vi "ClimberDeploy.vi"(8 "error in (no error)":errorcluster, 9 "Deploy/Retract":bool, 10 "Screw":dbl, 11 "ScissorClimber in":refnum<class "ScissorClimber.lvclass">) -> (0 "error out":errorcluster, 3 "ScissorClimber out":refnum<class "ScissorClimber.lvclass">)   [LabVIEW 2019, in "Climber.lvlib" / "ScissorClimber.lvclass"]
uses:
  ScissorClimber.lvclass
  Controls/DeployingStates.ctl
  <vilib>/Rock Robotics/WPI/ThirdParty/Phoenix-LabVIEW/Motor Controller/Controls/CTRE_Phoenix_MotorControl_ControlMode.ctl
  <vilib>/Rock Robotics/WPI/ThirdParty/Phoenix-LabVIEW/Motor Controller/Get/CTRE_Phoenix_MotorController_GetSelectedSensorData.vi
  Climber.lvclass
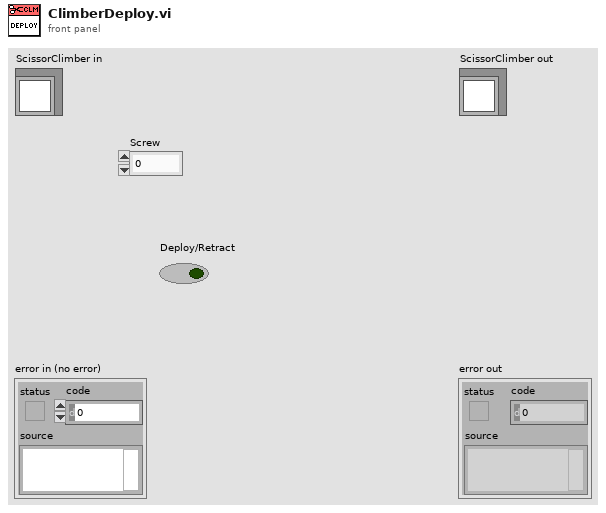
[diagram p1: front panel]
types:
  T1 = typedef "Climber.lvlib/Climber.lvclass/DeployingStates.ctl" = enum16{"Retract", "Manual Control", "Deploying", "Idle"}
  T2 = typedef "Climber.lvlib/Climber.lvclass/Screw Motor.ctl" = cluster{"Refnum Name":string, "CAN ID":u32, "I":dbl, "D":dbl, "P":dbl, "F":dbl, "Velocity":dbl, "Acceleration":dbl}
  T3 = typedef "CTRE_Phoenix_MotorControl_ControlMode.ctl" = u16
  T4 = typedef "WPI_MotorControlDeviceRef.ctl" = cluster{"DeviceStatus":errorcluster, "Type":T5, "PWM":cluster{"PWM Channel":T6, "DeadBand":T7}, "CAN":cluster{"Device Number":u8, "SetOutput VI Ref":variant, "GetOutput VI Ref":variant, "Enable VI Ref":variant, "Disable VI Ref":variant, "Data":variant}, "Invert":bool, "DIO PWM":cluster{"PWM \"Enable\" Channel":T6, "DIOChannel":T8, "PWM Rate":dbl}}
  T5 = typedef "WPI_MotorControlType.ctl" = enum16{"PWM", "CAN", "DIO PWM"}
  T6 = typedef "FPGA_DIOPWMChannel.ctl" = enum8{"PWM 0", "PWM 1", "PWM 2", "PWM 3", "PWM 4", "PWM 5", "PWM 6", "PWM 7", "PWM 8", "PWM 9", "PWM MXP 0", "PWM MXP 1", "PWM MXP 2", "PWM MXP 3", "PWM MXP 4", "PWM MXP 5", "PWM MXP 6", "PWM MXP 7", "PWM MXP 8", "PWM MXP 9", "Invalid"}
  T7 = typedef "WPI_PWMDeadband.ctl" = cluster{"Name":string, "maxPositivePwm":i32, "minPositivePwm":i32, "centerPwm":i32, "maxNegativePwm":i32, "minNegativePwm":i32, "angularRange":u16}
  T8 = typedef "FPGA_DIOChannel.ctl" = enum8{"DIO 0", "DIO 1", "DIO 2", "DIO 3", "DIO 4", "DIO 5", "DIO 6", "DIO 7", "DIO 8", "DIO 9", "DIO MXP 0", "DIO MXP 1", "DIO MXP 2", "DIO MXP 3", "DIO MXP 4", "DIO MXP 5", "DIO MXP 6", "DIO MXP 7", "DIO MXP 8", "DIO MXP 9", "DIO MXP 10", "DIO MXP 11", "DIO MXP 12", "DIO MXP 13", "DIO MXP 14", "DIO MXP 15", "SPI Port CS1", "SPI Port CS2", "SPI Port CS3", "SPI Port MISO", "SPI Port MOSI", "Invalid"}
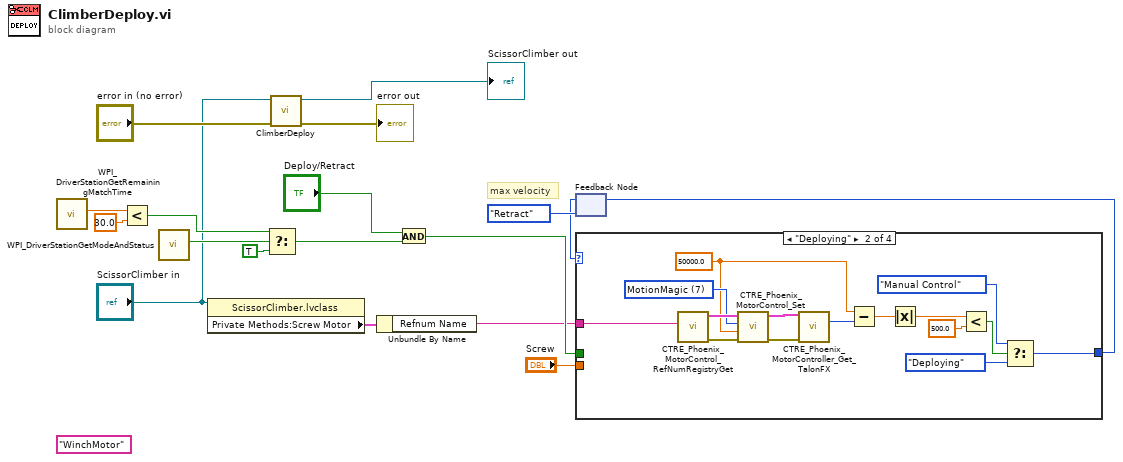
[diagram p0: block diagram]
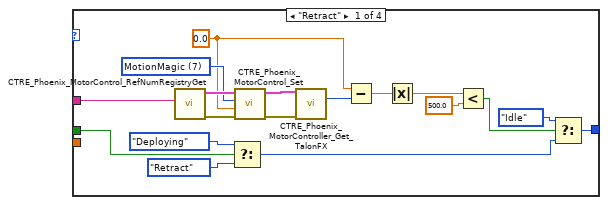
[diagram p2: hidden frame]
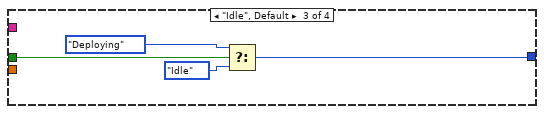
[diagram p3: hidden frame]
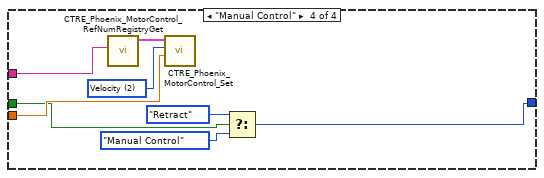
[diagram p4: hidden frame]
diagram:
  (unwired) "WinchMotor"
  # "max velocity"
  n1 = call <vilib>:"WPI_DriverStationGetRemainingMatchTime.vi"() -> ("Match Time(s)"=w15:sgl)  [unwired: 10 in, 1 out]
  n2 = Less?(x=w15, y=30.0) -> (x < y?=w11:bool)
  n3 = call <vilib>:"WPI_DriverStationGetModeAndStatus.vi"() -> ("FMS Attached"=w13:bool)  [unwired: 10 in, 1 out]
  n4 = property class="ScissorClimber.lvclass"(reference="ScissorClimber in") -> ("Private Methods:Screw Motor"=w2:T2)  [unwired: 1 in, 2 out]
  n5 = Select(t=w11, s=w13, f=TRUE) -> (s? t:f=w10:bool)
  n6 = call-parent "ClimberDeploy.vi"("error in (no error)"="error in (no error)", "Climber in"="ScissorClimber in") -> ("error out"=→"error out":errorcluster, "Climber out"=→"ScissorClimber out":refnum<class "ScissorClimber.lvclass">)  [unwired: 8 in]
  n7 = Unbundle By Name(w2) -> ("Refnum Name"=w1:string)
  n8 = And(x="Deploy/Retract", y=w10) -> (x .and. y?=w5:bool)
  n9 = feedback #1(DeployingStates."Retract") -> (w7:T1)
  n10 = case shown="\"Deploying\"" w7 {
    tunnel: [w23 w39 w53 w60] -> w6
    tunnel: w5 -> [w20 _ w52 w59]
    tunnel: "Screw" -> [_ _ _ w63]
    tunnel: w1 -> [w24 w38 _ w56]
    frame "Retract" {
      w31 = 0.0 ("Output")
      w34 = T3 7 items=["PercentOutput"=0, "Position"=1, "Velocity"=2, "Current"=3, "Follower"=5, "MotionProfile"=6, "MotionMagic"=7, "MotionProfileArc"=10, "Disabled"=15] ("Control Mode")
      n11 = call <vilib>:"CTRE_Phoenix_MotorControl_RefNumRegistryGet.vi"("refnum name"=w24) -> ("error out"=w36:errorcluster, "PhoenixMotorControlDevRef"=w35:T4)  [unwired: 9 in]
      n12 = Select(t=DeployingStates."Deploying", s=w20, f=DeployingStates."Retract") -> (s? t:f=w21:T1)
      n13 = call <vilib>:"CTRE_Phoenix_MotorControl_Set.vi"("error in (no error)"=w36, "Output"=w31, "Control Mode"=w34, "PhoenixMotorControlDevRef"=w35) -> ("error out"=w32:errorcluster, "PhoenixMotorControlDevRef"=w33:T4)  [unwired: 6 in]
      n14 = call-poly <vilib>:"CTRE_Phoenix_MotorController_Get_TalonFX.vi"("PhoenixMotorControlDevRef"=w33, "error in"=w32) -> ("Position (Raw Sensor Units)"=w30:i32)  [unwired: 10 in, 3 out]
      n15 = Subtract(x=w31, y=w30) -> (x-y=w29:dbl)
      n16 = Absolute Value(x=w29) -> (abs(x)=w28:dbl)
      n17 = Less?(x=w28, y=500.0) -> (x < y?=w26:bool)
      n18 = Select(t=DeployingStates."Idle", s=w26, f=w21) -> (s? t:f=w23:T1)
    }
    frame "Deploying" {
      w46 = 50000.0 ("Output")
      w49 = T3 7 items=["PercentOutput"=0, "Position"=1, "Velocity"=2, "Current"=3, "Follower"=5, "MotionProfile"=6, "MotionMagic"=7, "MotionProfileArc"=10, "Disabled"=15] ("Control Mode")
      n19 = call <vilib>:"CTRE_Phoenix_MotorControl_RefNumRegistryGet.vi"("refnum name"=w38) -> ("error out"=w51:errorcluster, "PhoenixMotorControlDevRef"=w50:T4)  [unwired: 9 in]
      n20 = call <vilib>:"CTRE_Phoenix_MotorControl_Set.vi"("error in (no error)"=w51, "Output"=w46, "Control Mode"=w49, "PhoenixMotorControlDevRef"=w50) -> ("error out"=w47:errorcluster, "PhoenixMotorControlDevRef"=w48:T4)  [unwired: 6 in]
      n21 = call-poly <vilib>:"CTRE_Phoenix_MotorController_Get_TalonFX.vi"("PhoenixMotorControlDevRef"=w48, "error in"=w47) -> ("Position (Raw Sensor Units)"=w37:i32)  [unwired: 10 in, 3 out]
      n22 = Subtract(x=w46, y=w37) -> (x-y=w45:dbl)
      n23 = Absolute Value(x=w45) -> (abs(x)=w44:dbl)
      n24 = Less?(x=w44, y=500.0) -> (x < y?=w42:bool)
      n25 = Select(t=DeployingStates."Manual Control", s=w42, f=DeployingStates."Deploying") -> (s? t:f=w39:T1)
    }
    frame "Idle", Default {
      n26 = Select(t=DeployingStates."Deploying", s=w52, f=DeployingStates."Idle") -> (s? t:f=w53:T1)
    }
    frame "Manual Control" {
      w61 = T3 2 items=["PercentOutput"=0, "Position"=1, "Velocity"=2, "Current"=3, "Follower"=5, "MotionProfile"=6, "MotionMagic"=7, "MotionProfileArc"=10, "Disabled"=15] ("Control Mode")
      n27 = call <vilib>:"CTRE_Phoenix_MotorControl_RefNumRegistryGet.vi"("refnum name"=w56) -> ("PhoenixMotorControlDevRef"=w62:T4)  [unwired: 9 in, 1 out]
      n28 = call <vilib>:"CTRE_Phoenix_MotorControl_Set.vi"("Output"=w63, "Control Mode"=w61, "PhoenixMotorControlDevRef"=w62) -> ()  [unwired: 7 in, 2 out]
      n29 = Select(t=DeployingStates."Retract", s=w59, f=DeployingStates."Manual Control") -> (s? t:f=w60:T1)
    }
  }
  n30 = feedback-in #1(w6) -> ()
